vi "S2C_FORNAX_Proc_ViperMsgAlarmScan.vi"(8 "Error In":errorcluster, 11 "Message":string) -> (0 "Error Out":errorcluster)   [LabVIEW 2015]
doc: "Extracts the Viper message from the DDS data stream."
uses:
  S2C_FORNAX_Proc_Globals.vi
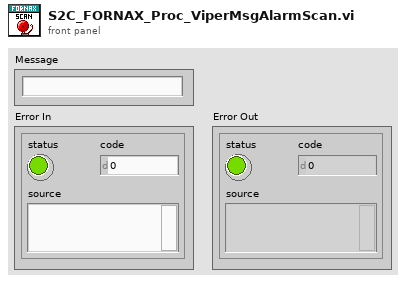
[diagram p1: front panel]
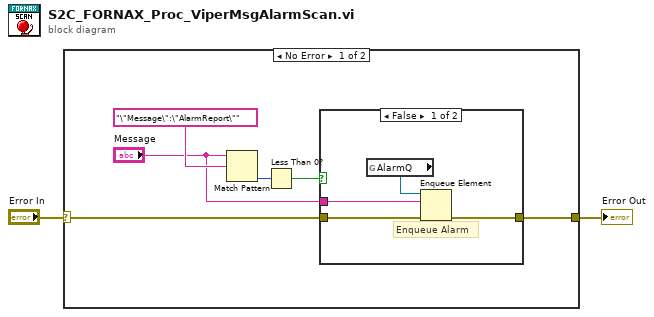
[diagram p0: block diagram]
diagram:
  n1 = case shown="No Error" "Error In" {
    selector: "Error In" -> [w6 w14]
    tunnel: [w4 w14] -> w1
    frame No Error {
      n2 = Match Pattern(string="Message", regular expression="\"Message\":\"AlarmReport\"") -> (offset past match=w7:i32)  [unwired: 1 in, 3 out]
      n3 = Less Than 0?(x=w7) -> (x < 0?=w5:bool)
      n4 = case shown="False" w5 {
        tunnel: w6 -> [w12 w13]
        tunnel: [w10 w13] -> w4
        tunnel: "Message" -> [w9 _]
        frame False {
          # "Enqueue Alarm"
          n5 = global read "S2C_FORNAX_Proc_Globals.vi" "AlarmQ"() -> (w11:refnum<queue>)
          n6 = Enqueue Element(queue=w11, element=w9, error in (no error)=w12) -> (error out=w10:errorcluster)  [unwired: 1 in, 2 out]
        }
        frame True {
        }
      }
    }
    frame Error {
    }
  }
  "Error Out" <- w1
